vi "Send Remote Message.vi"(5 "Target Task (None)":string, 7 "Target Node":string, 8 "error in (no error)":errorcluster, 9 "Message Type":string, 10 "Message":refnum<class "Message.lvclass">, 11 "Module in":refnum<class "Module.lvclass">) -> (0 "error out":errorcluster, 3 "Module out":refnum<class "Module.lvclass">)   [LabVIEW 2020, in "Volatus.lvlib" / "Module.lvclass"]
uses:
  Module.lvclass
  Module.lvclass/Module.ctl
  VolatusAPI/VolatusAPI.lvclass
  lv-protoc/LV-Proto/Message/Message.lvclass
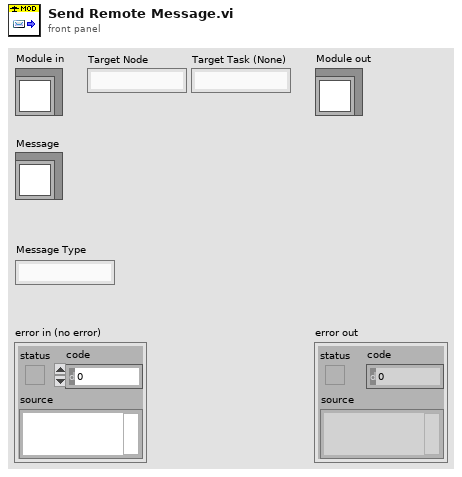
[diagram p1: front panel]
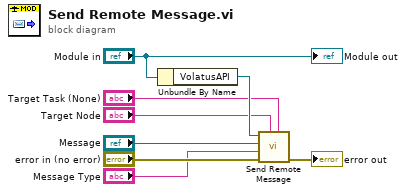
[diagram p0: block diagram]
diagram:
  n1 = Unbundle By Name("Module in") -> ("VolatusAPI"=w7:refnum<class "VolatusAPI.lvclass">)
  n2 = call "Send Remote Message.vi"("Target Task (None)"="Target Task (None)", "Target Node"="Target Node", "error in (no error)"="error in (no error)", "Message Type"="Message Type", "Message"="Message", "VolatusAPI in"=w7) -> ("error out"=→"error out":errorcluster)  [unwired: 4 in, 1 out]
  "Module out" <- "Module in"
